vi "ReadTiffPage_I16_text_res.vi"(0 "TIFF file":T2 {"BigTiff,Endian" items=["Big-Endian"=0, "Native"=1, "Little-Endian"=2, "BigTiff-Big-Endian"=256, "Bigtiff,Native"=257, "Biftiff,Littleendian"=258]}, 2 "IFDoffset":u64, 3 "error in":errorcluster) -> (4 "Pixelsize [µm]":cluster{"x":dbl, "y":dbl}, 6 "TIFF file out":T2 {"BigTiff,Endian" items=["Big-Endian"=0, "Native"=1, "Little-Endian"=2, "BigTiff-Big-Endian"=256, "Bigtiff,Native"=257, "Biftiff,Littleendian"=258]}, 7 "16-bit pixmap":i16[][](array[numeric]), 8 "string":string, 9 "Next offset":u64, 10 "error out":errorcluster)   [LabVIEW 2011]
uses:
  IFD.ctl
  GetTagValue_U64.vi
  GetTagValues_U8s.vi
  GetTagValue_Double.vi
panel:
  out "Byte-Reihenfolge (0:Big-Endian, Netzwerkreihenfolge)":T1(ring)=enum."native, host order"
  out "Bytes":u64
  out "Bits":u32
  out "BildOffset":u64
  out "Width":u64
  out "Length":u64
  out "Directory Entries":T3[](array[typedef])
  out "IFDs":u16
  # "seems to work!"
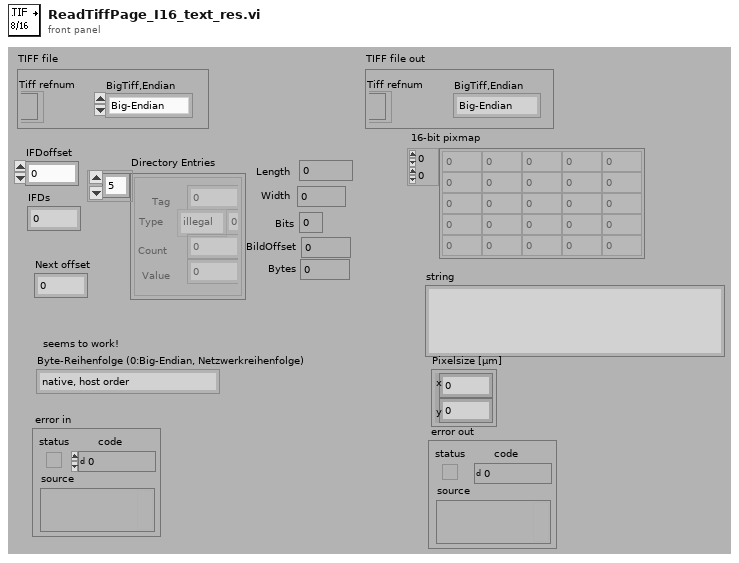
[diagram p1: front panel]
types:
  T1 = enum16{"big-endian, network order", "native, host order", "little-endian"}
  T2 = cluster{"Tiff refnum":refnum<file>, "BigTiff,Endian":u16}
  T3 = typedef "IFD.ctl" = cluster{"Tag":u16, "Type":enum16{"illegal", "Byte", "Ascii", "Short", "Long", "Rational", "SByte", "Undefined", "SShort", "SLong", "SRational 2xSLong", "Float 4byte", "Double 8Byte", "No13", "No14", "No15", "U64", "I64", "U64-IFD8"}, "Count":u64, "Value":u64}
  T4 = cluster{"Tag":u16, "Type":enum16{"illegal", "Byte", "Ascii", "Short", "Long", "Rational", "SByte", "Undefined", "SShort", "SLong", "SRational 2xSLong", "Float 4byte", "Double 8Byte"}, "Count":u32, "Value":u32}
  T5 = cluster{"Tag":u16, "Type":enum16{"illegal", "Byte", "Ascii", "Short", "Long", "Rational", "SByte", "Undefined", "SShort", "SLong", "SRational 2xSLong", "Float 4byte", "Double 8Byte"}, "Count":u32, "Value":u32}[]
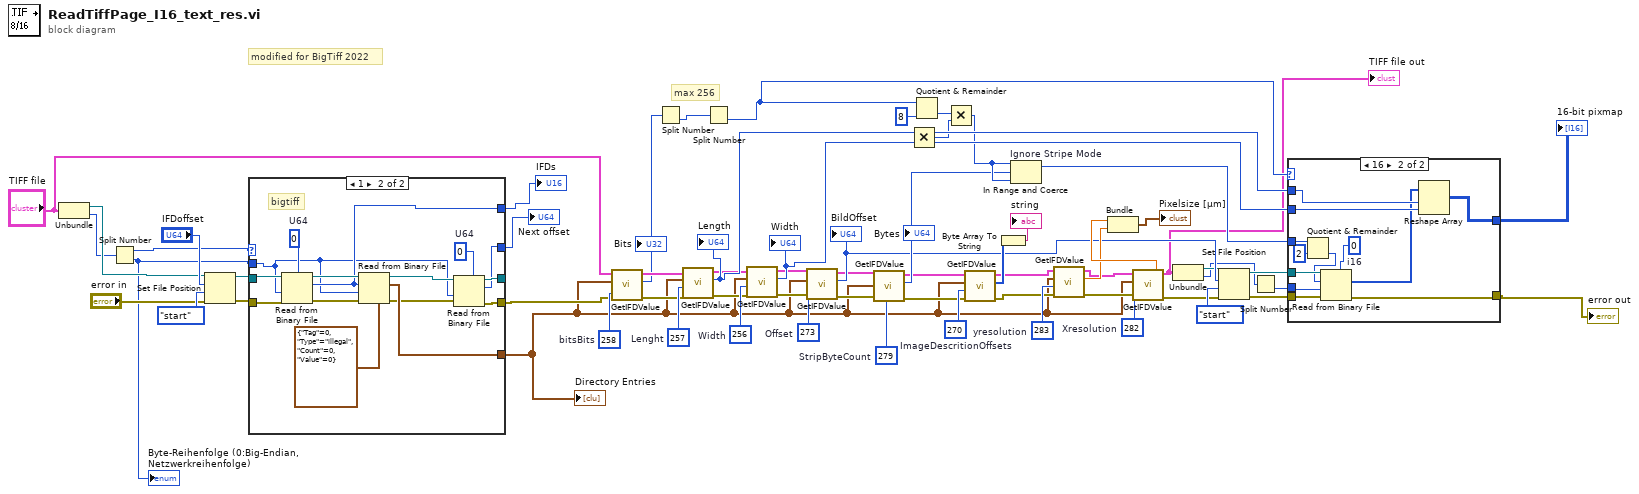
[diagram p0: block diagram]
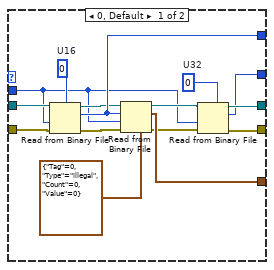
[diagram p2: hidden frame]
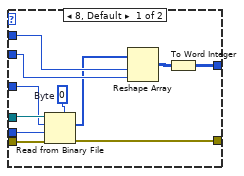
[diagram p3: hidden frame]
diagram:
  w42 = u16 283  # yresolution
  w44 = u16 282  # Xresolution
  w39 = u16 270  # ImageDescritionOffsets
  w53 = u16 256  # Width
  w60 = u16 258  # bitsBits
  w52 = u16 279  # StripByteCount
  w55 = u16 257  # Lenght
  w54 = u16 273  # Offset
  # "modified for BigTiff 2022"
  # "max 256"
  n1 = Unbundle("TIFF file") -> ("Tiff refnum"=w56:refnum<file>, "BigTiff,Endian"=w14:u16)
  n2 = Split Number(x=w14) -> (hi(x)=w3:u8, lo(x)=w4:u8)
  "Byte-Reihenfolge (0:Big-Endian, Netzwerkreihenfolge)" <- w4
  n3 = Set File Position(offset (in bytes) (0)="IFDoffset", refnum=w56, from (0:start)=enum16{"start", "end", "current"}."start" ("pos mode (0:2)"), error in="error in") -> (refnum out=w5:refnum<file>, error out=w8:errorcluster)
  n4 = case shown="1" w3 {
    tunnel: [w77 w87] -> w1
    tunnel: w8 -> [w76 w89]
    tunnel: w5 -> [w75 w88]
    tunnel: [w68 w82] -> _
    tunnel: [w67 w84] -> w7
    tunnel: [w72 w86] -> w6
    tunnel: w4 -> [w64 w81]
    tunnel: [w66 w79] -> w2
    frame 0, Default {
      w65 = u32 0  # U32
      w78 = u16 0  # U16
      n5 = Read from Binary File(5:w78, 8:w76, 9:w64, 11:w75) -> (0:w73:errorcluster, 2:w77:u16, 3:w74:refnum<file>)  [unwired: 3 out]
      n6 = Read from Binary File(5:T4 {"Tag"=0, "Type"=enum."illegal", "Count"=0, "Value"=0} ("Cluster"), 8:w73, 9:w64, 10:w77, 11:w74) -> (0:w70:errorcluster, 2:w72:T5, 3:w69:refnum<file>)  [unwired: 2 out]
      n7 = Read from Binary File(5:w65, 8:w70, 9:w64, 11:w69) -> (0:w67:errorcluster, 2:w66:u32, 3:w68:refnum<file>)  [unwired: 3 out]
    }
    frame 1 {
      w80 = u64 0  # U64
      w93 = u64 0  # U64
      # "bigtiff"
      n8 = Read from Binary File(5:w93, 8:w89, 9:w81, 11:w88) -> (0:w91:errorcluster, 2:w87:u64, 3:w92:refnum<file>)  [unwired: 3 out]
      n9 = Read from Binary File(5:T3 {"Tag"=0, "Type"=enum."illegal", "Count"=0, "Value"=0} ("Cluster"), 8:w91, 9:w81, 10:w87, 11:w92) -> (0:w85:errorcluster, 2:w86:T3[], 3:w83:refnum<file>)  [unwired: 2 out]
      n10 = Read from Binary File(5:w80, 8:w85, 9:w81, 11:w83) -> (0:w84:errorcluster, 2:w79:u64, 3:w82:refnum<file>)  [unwired: 3 out]
    }
  }
  "IFDs" <- w1
  "Directory Entries" <- w6
  "Next offset" <- w2
  n11 = call-poly "GetIFDValue.vi"("error in (no error)"=w7, "Tag Code"=w60, "Directory Entries"=w6, "TIFF file"="TIFF file") -> ("error out"=w35:errorcluster, "Single Value"=w12:u64, "TIFF file out"=w37:T2)  [unwired: 3 out]
  "Bits" <- w12
  n12 = Split Number(x=w12) -> (lo(x)=w13:u32)  [unwired: 1 out]
  n13 = call-poly "GetIFDValue.vi"("error in (no error)"=w35, "Tag Code"=w55, "Directory Entries"=w6, "TIFF file"=w37) -> ("error out"=w34:errorcluster, "Single Value"=w51:u64, "TIFF file out"=w36:T2)  [unwired: 3 out]
  "Length" <- w51
  n14 = Split Number(x=w13) -> (lo(x)=w11:u16)  [unwired: 1 out]
  n15 = call-poly "GetIFDValue.vi"("error in (no error)"=w34, "Tag Code"=w53, "Directory Entries"=w6, "TIFF file"=w36) -> ("error out"=w30:errorcluster, "Single Value"=w50:u64, "TIFF file out"=w32:T2)  [unwired: 3 out]
  "Width" <- w50
  n16 = call-poly "GetIFDValue.vi"("error in (no error)"=w30, "Tag Code"=w54, "Directory Entries"=w6, "TIFF file"=w32) -> ("error out"=w29:errorcluster, "Single Value"=w33:u64, "TIFF file out"=w31:T2)  [unwired: 3 out]
  "BildOffset" <- w33
  n17 = call-poly "GetIFDValue.vi"("error in (no error)"=w29, "Tag Code"=w52, "Directory Entries"=w6, "TIFF file"=w31) -> ("error out"=w28:errorcluster, "Single Value"=w45:u64, "TIFF file out"=w24:T2)  [unwired: 3 out]
  "Bytes" <- w45
  n18 = Multiply(x=w51, y=w50) -> (x*y=w48:u64)
  n19 = Quotient & Remainder(x=w11, y=u32 8) -> (floor(x/y)=w47:u32)  [unwired: 1 out]
  n20 = Multiply(x=w47, y=w48) -> (x*y=w46:u64)
  n21 = call-poly "GetIFDValue.vi"("error in (no error)"=w28, "Tag Code"=w39, "Directory Entries"=w6, "TIFF file"=w24) -> ("error out"=w27:errorcluster, "Byte array"=w38:u8[], "TIFF file out"=w22:T2)  [unwired: 3 out]
  n22 = Byte Array To String(unsigned byte array=w38) -> (string=→"string":string)
  n23 = In Range and Coerce "Ignore Stripe Mode"(upper limit=w46, x=w45, lower limit=w46) -> (coerced(x)=w16:u64)  [unwired: 1 out]
  n24 = call-poly "GetIFDValue.vi"("error in (no error)"=w27, "Tag Code"=w42, "Directory Entries"=w6, "TIFF file"=w22) -> ("error out"=w26:errorcluster, "Value"=w41:dbl, "TIFF file out"=w21:T2)  [unwired: 3 out]
  n25 = call-poly "GetIFDValue.vi"("error in (no error)"=w26, "Tag Code"=w44, "Directory Entries"=w6, "TIFF file"=w21) -> ("error out"=w25:errorcluster, "Value"=w43:dbl, "TIFF file out"=w10:T2)  [unwired: 3 out]
  "TIFF file out" <- w10
  n26 = Bundle("Value"=w43, "Value"=w41) -> (→"Pixelsize [µm]":cluster{"Value":dbl, "Value":dbl})  [unwired: 1 out]
  n27 = Unbundle(w10) -> ("Tiff refnum"=w20:refnum<file>, "BigTiff,Endian"=w15:u16)
  n28 = Set File Position(offset (in bytes) (0)=w33, refnum=w20, from (0:start)=enum16{"start", "end", "current"}."start" ("pos mode (0:2)"), error in=w25) -> (refnum out=w19:refnum<file>, error out=w18:errorcluster)
  n29 = Split Number(x=w15) -> (lo(x)=w9:u8)  [unwired: 1 out]
  n30 = case shown="16" w11 {
    tunnel: w51 -> [w104 w116]
    tunnel: w50 -> [w103 w115]
    tunnel: [w94 w114] -> w59
    tunnel: w19 -> [w101 w113]
    tunnel: w18 -> [w100 w112]
    tunnel: [w99 w106] -> w17
    tunnel: w16 -> [w96 w110]
    tunnel: w9 -> [w95 w111]
    frame 8, Default {
      w97 = u8 0  # Byte
      n31 = Read from Binary File(5:w97, 8:w100, 9:w95, 10:w96, 11:w101) -> (0:w99:errorcluster, 2:w98:u8[])  [unwired: 3 out]
      n32 = Reshape Array(w98, w104, w103) -> (w102:u8[][])
      n33 = To Word Integer(number=w102) -> (16bit integer=w94:i16[][])
    }
    frame 16 {
      w107 = i16 0  # i16
      n34 = Quotient & Remainder(x=w110, y=u32 2) -> (floor(x/y)=w108:u64)  [unwired: 1 out]
      n35 = Read from Binary File(5:w107, 8:w112, 9:w111, 10:w108, 11:w113) -> (0:w106:errorcluster, 2:w105:i16[])  [unwired: 3 out]
      n36 = Reshape Array(w105, w116, w115) -> (w114:i16[][])
    }
  }
  "error out" <- w17
  "16-bit pixmap" <- w59
